vi "GUI.vi"() -> ()   [LabVIEW 2015]
doc: "The myRIO Project template acquires acceleration data from the onboard accelerometer and displays the changes of acceleration values in a waveform chart."
uses:
  Labview/Kinect Project/Kinect Project/subVIs/Log Level Control.ctl
  Labview/Kinect Project/Kinect Project/subVIs/Video Resolution Control.ctl
  Labview/Kinect Project/Kinect Project/subVIs/Video Format Control.ctl
  Labview/Kinect Project/Kinect Project/subVIs/Depth Format Control.ctl
  Labview/Kinect Project/Kinect Project/subVIs/Depth Resolution Control.ctl
  Labview/Kinect Project/Kinect Project/subVIs/Led Control.ctl
panel:
  out "Start angle":dbl
  in  "Ring":u16(ring)
  out "Hazard location":dbl[](array[numeric])
  out "# of targets chosen":dbl
  out "Tab indicator":string
  in  "Map Displays":enum32{"Display map", "Obsticle map"}(tab)
  out "Display map":u16[][](array[ring])
  in  "Obsticle map":u16[][](array[ring])
  in  "Robot information":enum32{"Robot info", "Status updates"}(tab)
  out "Paused LED":bool
  out "Robot angle":dbl
  out "Robot location (grid)":dbl[](array[numeric])
  out "Target location":dbl[](array[numeric])
  out "Route":dbl[][](array[numeric])
  out "Robot location (cm)":dbl[](array[numeric])
  in  "Pause":bool
  in  "stop":bool
  out "Map key words":string[](array[string])
  out "Map key":u16[](array[ring])
  out "Waitning for user input LED":bool
  out "Executing route LED":bool
  out "Slecting target LED":bool
  out "Altering amp LED":bool
  out "Scanning LED":bool
  out "Initializing LED":bool
  in  "Options and instructions":T1(tab)
  out "Initialize map LED":bool
  in  "Robot starting angle":dbl
  in  "Robot starting location":dbl[](array[numeric])
  in  "Load":bool
  in  "Start":bool
  in  "Angle to scan around":dbl
  in  "Scan or move toggle":bool
  in  "Start scan or move button":bool
  out "Scan or move":bool
  in  "Run auto correct":bool
  out "Auto correct Led":bool
  in  "Alter map button":bool
  out "Alter map LED":bool
  out "To many targets":bool
  in  "Chose location button":bool
  in  "Chose location switch":bool
  out "Calulated target location":dbl[](array[numeric])
  out "Chose location LED":bool
  out "Kinect Handle":i64
  out "Video Handle out":i64
  out "Object location":dbl[][](array[numeric])
  out "p":dbl
  out "Centre location":dbl[](array[numeric])
  out "Map dimensions":dbl[](array[numeric])
  # "The text on the left indicates which \ntab you should be on"
  # "On the right is the robots location on the grid and\nin cm from the top left corner of the map"
  # "The angle the robot is facing is displayed on the right. An angle of 0 \nis relative to north on the map, 90 is east, 180 is south and 270 is west"
  # "The destiniation on the grid that the robot is trying to reach is \ndisplayed in the box Target location and the route it will take \ndisplayed in Route"
  # "If you wish to stop the program from running press the button in\nthe top right of the screen or the button to the right. To pause the \nprogram after its current task use the toggle switch to the left"
  # "When paused light will be on"
  # "The lights below indicate what task the \nrobot is currently completing"
  # "Below is the key for the map"
  # "Initializing"
  # "Scanning for hazards and obsticles"
  # "Altering map"
  # "Selecting target location"
  # "Executing route"
  # "Waiting for user input"
  # "When this light is on you will need to select the initilization mode"
  # "Use the switch on the left to select wether you want to start from a new \npredefined map or wether you want to start from the last saved map. It is \nkey that if conection was lost and restablished that you start from loading \nthe last saved map"
  # "If you are starting from the a new map type in the starting location of \nthe robot. Remeber that the angle is relative to NSEW on the map with \nan angle of 0 being North"
  # "Once you are happy with your selection press the start button to the left \nto start the robot moving."
  # "When this light is on you can choose wether to move to another \npoint or scan at the robots current location"
  # "Using the toggle switch to the right you will be able to chose \nwether you want to scan 180 degree around the robots current \nloation after which you can adjust the map and chose the next \nlocation to move to or wether you would like the robot just move \nto a location before which you can alter the map if need be"
  # "If you decide to scan you can alter the angle that the DaNI will scan\naround. The angle will be defaulted to the DaNI's current location"
  # "Once you are have decided on wether to move or scan using \nthe toggle swtich, press the button on the right to select your \nchosen option"
  # "When this light is on you will be able to alter the map for any errors.\nYou can manualy make changes but this should only be done at this \nstage and on the obsticle map"
  # "If you would like the program to run an autocorrect on the map press\nthe button to the right. If the green light is on autocorrect is running \nso don't change anything on the map as it will not be saved."
  # "Once you are happy with the changes press the button on the left and\nthe changes will be saved and the program will continue executing"
  # "When this light is on you will need to select the location to use.\nIf the light on the right flashes too many or not enough locations\nwhere selected"
  # "Use this screen to decide wether to use the target location calulated \nby the program or select your own target location. Once the taget \nlocation has been set a route will be calulated and the robot will \nmove to this location"
  # "Use the switch on the left to select wether to use the calculated\nlocation or use your own. To select your own select it on the map \nby changing the square Dark blue. Only select one square or it will \nnot be accepted"
  # "Once you are happy with the chosen location press the button \non the left to continue"
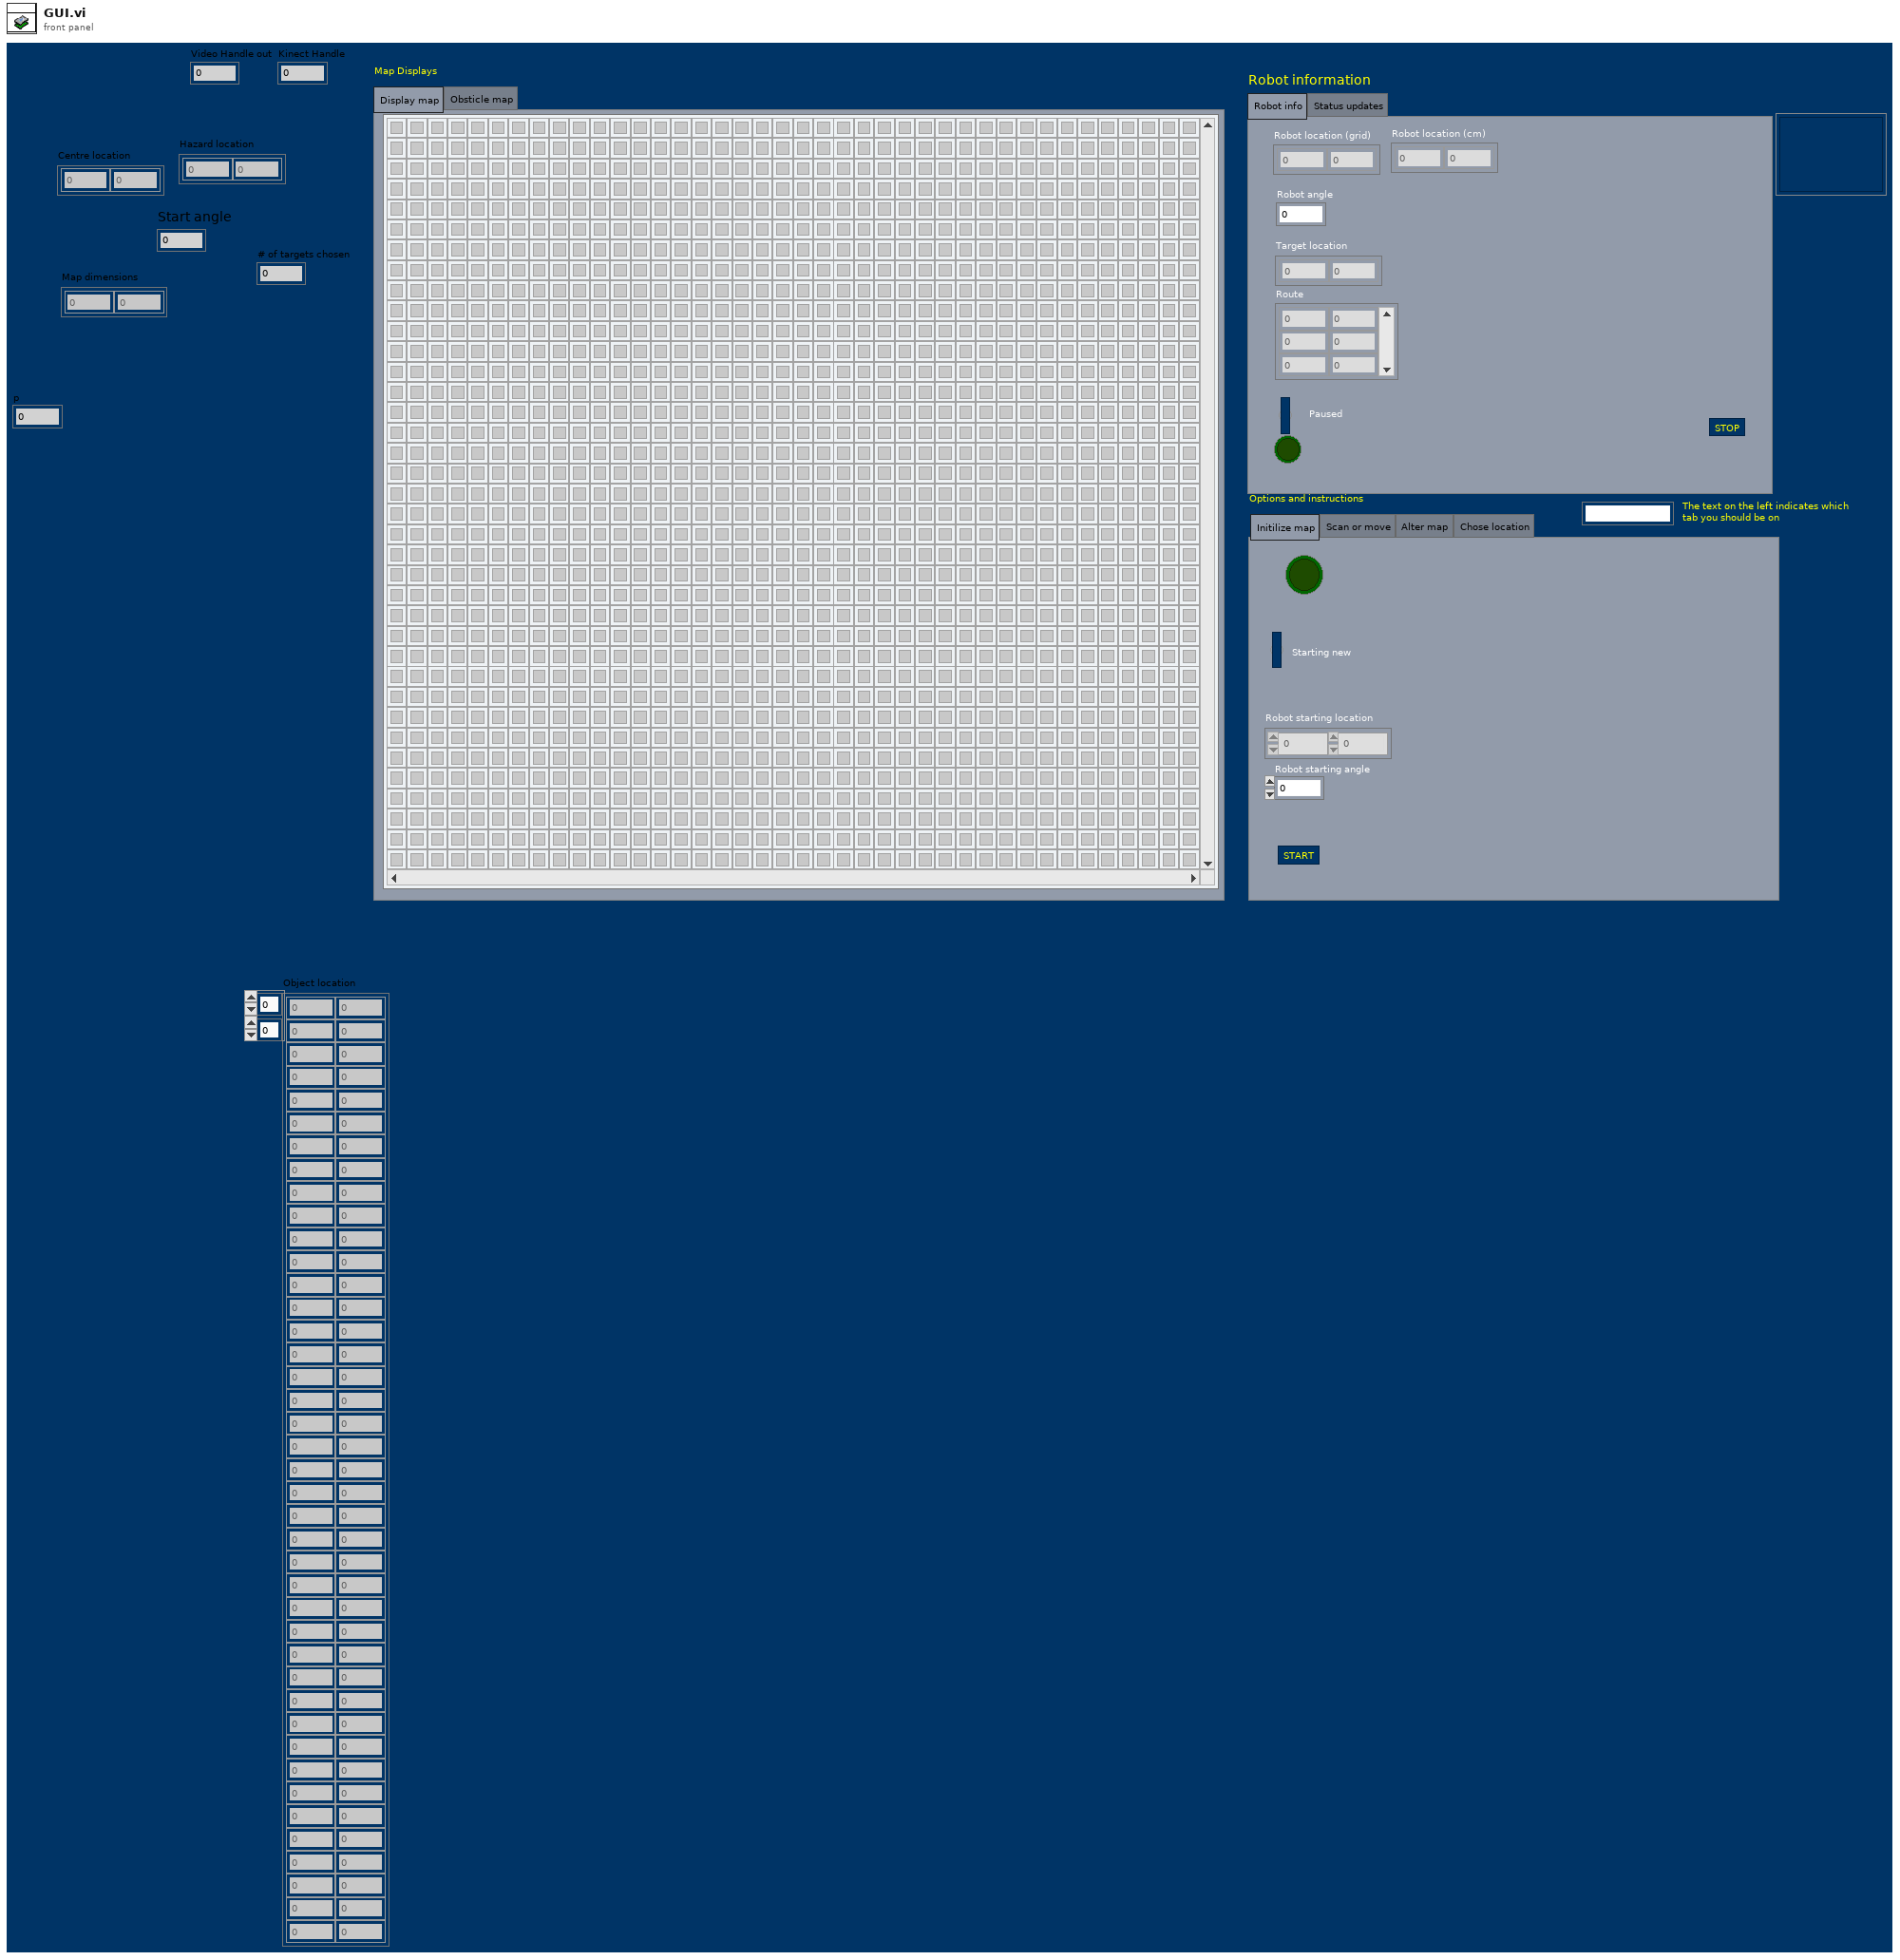
[diagram p1: front panel]
types:
  T1 = enum32{"Initilize map", "Scan or move", "Alter map", "Chose location"}
  T2 = typedef "Led Control.ctl" = enum32{"LED_OFF", "LED_GREEN", "LED_RED", "LED_YELLOW", "LED_BLINK_GREEN", "LED_BLINK_GREEN2", "LED_BLINK_RED_YELLOW"}
  T3 = typedef "Video Resolution Control.ctl" = enum32{"FREENECT_RESOLUTION_LOW", "FREENECT_RESOLUTION_MEDIUM", "FREENECT_RESOLUTION_HIGH"}
  T4 = typedef "Video Format Control.ctl" = enum32{"FREENECT_VIDEO_RGB", "FREENECT_VIDEO_BAYER", "FREENECT_VIDEO_IR_8BIT", "FREENECT_VIDEO_IR_10BIT", "FREENECT_VIDEO_IR_10BIT_PACKED", "FREENECT_VIDEO_YUV_RGB", "FREENECT_VIDEO_YUV_RAW"}
  T5 = typedef "Depth Format Control.ctl" = enum32{"FREENECT_DEPTH_11BIT", "FREENECT_DEPTH_10BIT", "FREENECT_DEPTH_11BIT_PACKED", "FREENECT_DEPTH_10BIT_PACKED", "FREENECT_DEPTH_REGISTERED", "FREENECT_DEPTH_MM"}
  T6 = typedef "Depth Resolution Control.ctl" = enum16{"FREENECT_RESOLUTION_TINY", "FREENECT_RESOLUTION_LOW", "FREENECT_RESOLUTION_MEDIUM"}
  T7 = cluster{"Video Resolution":T3, "Video Format":T4, "Depth Format":T5, "Depth Resolution":T6}
  T8 = typedef "Log Level Control.ctl" = enum32{"FREENECT_LOG_FATAL", "FREENECT_LOG_ERROR", "FREENECT_LOG_WARNING", "FREENECT_LOG_NOTICE", "FREENECT_LOG_INFO", "FREENECT_LOG_DEBUG", "FREENECT_LOG_SPEW", "FREENECT_LOG_FLOOD"}
  T9 = cluster{"Hue Range":cluster{"Lower value":i32, "Upper value":i32}, "Sat Range":cluster{"Lower value":i32, "Upper value":i32}, "Luma Range":cluster{"Lower value":i32, "Upper value":i32}}
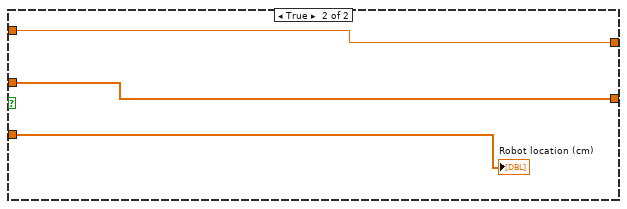
[diagram p2: hidden frame]
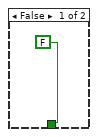
[diagram p5: hidden frame]
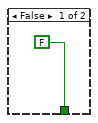
[diagram p6: hidden frame]
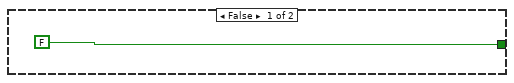
[diagram p8: hidden frame]
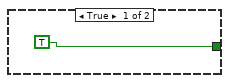
[diagram p9: hidden frame]
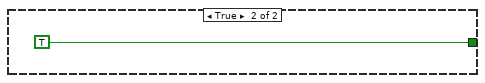
[diagram p10: hidden frame]
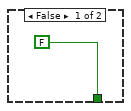
[diagram p12: hidden frame]
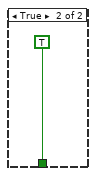
[diagram p13: hidden frame]
diagram:
  n1 = flat-sequence {
    frame #0 {
      n2 = flat-sequence {
        tunnel: [w7] -> w2
        tunnel: [w7] -> w1
        tunnel: w2 -> [w15]
        tunnel: w1 -> [w14]
        frame #0 {
          w3 = FALSE
          n3 = local write "Waitning for user input LED"(w3) -> ()
          n4 = local write "Executing route LED"(w3) -> ()
          n5 = local write "Initializing LED"(w3) -> ()
          n6 = local write "Paused LED"(w3) -> ()
          n7 = local write "Altering amp LED"(w3) -> ()
          n8 = local write "Slecting target LED"(w3) -> ()
          n9 = local write "Scanning LED"(w3) -> ()
          "Map key" <- i32[] [0, 1, 2, 4, 6, 3, 7, 8, 5]
          "Map key words" <- string[] ["Empty area", "Obsticle", "Unexplored area", "Robot location", "Robots front", "Target location", "Route", "Hazard", "Black box"]
        }
        frame #1 {
          w6 = FALSE
          n10 = while {
            tunnel: ["Load"] -> w7
            stop <- "Start" stop-if-true
            w10 = TRUE
            "Tab indicator" <- "Initialize map tab"
            "Initialize map LED" <- w10
            "Initializing LED" <- w10
          }
          n11 = local write "Auto correct Led"(w6) -> ()
          n12 = local write "Chose location LED"(w6) -> ()
          n13 = local write "Alter map LED"(w6) -> ()
          n14 = local write "Robot location (cm)"(dbl[] [0.0, 0.0]) -> ()
          n15 = local write "Route"(i32[][] []) -> ()
          n16 = local write "Scan or move"(w6) -> ()
        }
        frame #2 {
          n17 = call "Inizialize map.vi"("Boolean"=w14) -> ("Map dimesions"=→"Map dimensions":dbl[], "Map initialize"=w17:dbl[][], "Robot start location"=w18:dbl[], "Robot actual location"=w20:dbl[], "Robot angle"=w22:dbl)  [unwired: 6 in]
          n18 = local write "Obsticle map"(w17) -> ()
          n19 = case shown="False" w15 {
            tunnel: w18 -> [_ w43]
            tunnel: ["Robot starting location" w43] -> w19
            tunnel: w20 -> [_ w41]
            tunnel: ["Robot starting angle" w42] -> w21
            tunnel: w22 -> [_ w42]
            frame False {
              w30 = 2.5
              w35 = 5
              n20 = Index Array(array="Robot starting location", index #1=0, index #2=1) -> (element #1=w37:dbl, element #2=w36:dbl)
              n21 = Multiply(x=w37, y=w35) -> (x*y=w33:dbl)
              n22 = Multiply(x=w36, y=w35) -> (x*y=w34:dbl)
              n23 = Add(x=w33, y=w30) -> (x+y=w25:dbl)
              n24 = Add(x=w34, y=w30) -> (x+y=w26:dbl)
              n25 = local read "Robot location (cm)"() -> (w27:dbl[])
              n26 = Replace Array Subset(array=w27, new element #1=w25, index #1=0, new element #2=w26, index #2=1) -> (w28:dbl[])
              n27 = local write "Robot location (cm)"(w28) -> ()
            }
            frame True {
              "Robot location (cm)" <- w41
            }
          }
          "Robot location (grid)" <- w19
          "Robot angle" <- w21
          n28 = local write "Initialize map LED"(FALSE) -> ()
          n29 = local write "Tab indicator"("Any") -> ()
        }
        frame #3 {
          n30 = call "Initialize IMU.vi"() -> ()  [unwired: 12 in]
          n31 = call "LED control.vi"("RED/green"="Green") -> ()  [unwired: 11 in]
        }
        frame #4 {
          n32 = call "Initialize kinect systems.vi"("Video and Depth config"=T7 {"Video Resolution"=enum."FREENECT_RESOLUTION_MEDIUM", "Video Format"=enum."FREENECT_VIDEO_RGB", "Depth Format"=enum."FREENECT_DEPTH_11BIT", "Depth Resolution"=enum."FREENECT_RESOLUTION_LOW"} ("Video & Depth Config"), "Led Option"=Led_Control."LED_OFF", "tilt degree"=-15 ("Tilt degree"), "Log Level"=Log_Level_Control."FREENECT_LOG_FATAL") -> ("Kinect Handle"=→"Kinect Handle":i64, "Video Handle out"=→"Video Handle out":i64)  [unwired: 4 in, 2 out]
        }
        frame #5 {
          n33 = local read "Robot location (cm)"() -> (w53:dbl[])
          n34 = local read "Robot angle"() -> (w54:dbl)
          n35 = local read "Obsticle map"() -> (w52:u16[][])
          n36 = call "Update robot location and direction.vi"("Map input"=w52, "Actual robot location"=w53, "Robot angle"=w54) -> ("Map Output"=→"Display map":dbl[][], "Centre location"=→"Centre location":dbl[])  [unwired: 6 in]
          n37 = local write "Initializing LED"(FALSE) -> ()
        }
        frame #6 {
          n38 = while {
            stop <- w57 stop-if-true
            n39 = local read "Pause"() -> (w57:bool)
            n40 = local write "Paused LED"(TRUE) -> ()
          }
        }
      }
    }
    frame #1 {
      n41 = while {
        stop <- "stop" stop-if-true
        n42 = flat-sequence {
          tunnel: [w63] -> w60
          tunnel: w60 -> [w72]
          tunnel: [w72] -> w59
          tunnel: w59 -> [w74]
          frame #0 {
            n43 = local read "Robot angle"() -> (w62:dbl)
            n44 = local write "Angle to scan around"(w62) -> ()
          }
          frame #1 {
            n45 = while {
              tunnel: ["Scan or move toggle"] -> w63
              stop <- "Start scan or move button" stop-if-true
              n46 = local write "Paused LED"(FALSE) -> ()
              n47 = local write "Tab indicator"("Scan or move") -> ()
              n48 = call "LED control.vi"("RED/green"="Red") -> ()  [unwired: 11 in]
              "Scan or move" <- TRUE
              "Waitning for user input LED" <- TRUE
            }
          }
          frame #2 {
            n49 = call "LED control.vi"("RED/green"="Green") -> ()  [unwired: 11 in]
          }
          frame #3 {
            w73 = FALSE
            n50 = case shown="True" w74 {
              frame False {
              }
              frame True {
                n51 = flat-sequence {
                  frame #0 {
                    n52 = local read "Robot angle"() -> (w77:dbl)
                    n53 = call "Turning control.vi"("Robot angle"=w77, "Angle to move to"="Angle to scan around") -> ("Final Robot angle"=w76:dbl)  [unwired: 8 in]
                    n54 = local write "Angle to scan around"(w76) -> ()
                  }
                  frame #1 {
                    n55 = local read "Robot angle"() -> (w81:dbl)
                    n56 = call "correct angle.vi"("Robot angle"=w81, "Angle moved"=-90.0) -> ("Final angle"=w80:dbl)  [unwired: 9 in]
                    n57 = call "Turning control.vi"("Robot angle"=w81, "Angle to move to"=w80) -> ("Final Robot angle"=w79:dbl)  [unwired: 8 in]
                    "Start angle" <- w79
                    n58 = local write "Robot angle"(w79) -> ()
                    "Scanning LED" <- TRUE
                  }
                  frame #2 {
                    n59 = while {
                      stop <- w84 stop-if-true
                      n60 = flat-sequence {
                        tunnel: [w93] -> w87
                        tunnel: w87 -> [w94]
                        tunnel: [w94] -> w86
                        tunnel: w86 -> [w97]
                        tunnel: [w102] -> w88
                        tunnel: w88 -> [w108]
                        tunnel: [w113] -> _
                        tunnel: [w113] -> w85
                        tunnel: w85 -> [w121]
                        tunnel: [w122] -> w84
                        frame #0 {
                          n61 = local read "Robot location (cm)"() -> (w92:dbl[])
                          n62 = local read "Robot angle"() -> (w93:dbl)
                          n63 = call "Kinect Depth Controler.vi"("Angle"=w93, "Robot Location"=w92) -> ("p"=→"p":dbl, "Object location"=→"Object location":dbl[][])  [unwired: 7 in, 1 out]
                          n64 = local write "Paused LED"(FALSE) -> ()
                        }
                        frame #1 {
                        }
                        frame #2 {
                          n65 = local read "Obsticle map"() -> (w96:u16[][])
                          n66 = local read "Object location"() -> (w95:dbl[][])
                          n67 = local read "Robot location (grid)"() -> (w99:dbl[])
                          n68 = local read "p"() -> (w98:dbl)
                          n69 = call "Update obsticles.vi"("angle input"=w97, "Robot Location"=w99, "p"=w98, "Map Input"=w96, "Object location"=w95) -> ("Map output"=w100:dbl[][])  [unwired: 6 in]
                          n70 = local write "Obsticle map"(w100) -> ()
                        }
                        frame #3 {
                          n71 = local read "Robot location (cm)"() -> (w106:dbl[])
                          n72 = local read "Robot angle"() -> (w105:dbl)
                          n73 = call "Kinect Video Controller.vi"("HSL Ranges"=T9 {"Hue Range"={"Lower value"=200, "Upper value"=254}, "Sat Range"={"Lower value"=190, "Upper value"=254}, "Luma Range"={"Lower value"=0, "Upper value"=140}}, "Robot angle"=w105, "robot location"=w106) -> ("y"=w103:dbl, "x"=w101:dbl, "Hazard location"=→"Hazard location":dbl[])  [unwired: 6 in]
                          n74 = call "Validate hazard.vi"("y"=w103, "x"=w101) -> ("Valid"=w102:bool)  [unwired: 9 in]
                        }
                        frame #4 {
                          n75 = case shown="True" w108 {
                            frame False {
                            }
                            frame True {
                              n76 = local read "Obsticle map"() -> (w111:u16[][])
                              n77 = local read "Hazard location"() -> (w110:dbl[])
                              n78 = call "Update Hazards.vi"("Map Input"=w111, "Hazard location"=w110) -> ("Map Output"=w109:dbl[][])  [unwired: 9 in]
                              n79 = local write "Obsticle map"(w109) -> ()
                            }
                          }
                        }
                        frame #5 {
                          n80 = local read "Robot angle"() -> (w114:dbl)
                          n81 = call "turning.vi"("Turn time"=110, "clock anticlock"="Clock") -> ("angle moved"=w115:dbl)  [unwired: 9 in]
                          n82 = call "correct angle.vi"("Robot angle"=w114, "Angle moved"=w115) -> ("Final angle"=w113:dbl)  [unwired: 9 in]
                          n83 = local write "Robot angle"(w113) -> ()
                        }
                        frame #6 {
                          w117 = 5
                          n84 = local read "Start angle"() -> (w126:dbl)
                          n85 = call "correct angle.vi"("Robot angle"=w126, "Angle moved"=180) -> ("Final angle"=w120:dbl)  [unwired: 9 in]
                          n86 = Add(x=w120, y=w117) -> (x+y=w119:dbl)
                          n87 = Subtract(x=w120, y=w117) -> (x-y=w118:dbl)
                          n88 = Less Or Equal?(x=w121, y=w119) -> (x <= y?=w123:bool)
                          n89 = Greater Or Equal?(x=w121, y=w118) -> (x >= y?=w124:bool)
                          n90 = case shown="True" w124 {
                            tunnel: w123 -> [_ w129]
                            tunnel: [FALSE w128] -> w122
                            frame False {
                            }
                            frame True {
                              n91 = case shown="True" w129 {
                                tunnel: [FALSE TRUE] -> w128
                                frame False {
                                }
                                frame True {
                                }
                              }
                            }
                          }
                        }
                        frame #7 {
                          n92 = while {
                            stop <- w132 stop-if-true
                            n93 = local read "Pause"() -> (w132:bool)
                            n94 = local write "Paused LED"(FALSE) -> ()
                          }
                        }
                      }
                    }
                  }
                  frame #3 {
                    n95 = local read "Robot angle"() -> (w135:dbl)
                    n96 = call "correct angle.vi"("Robot angle"=w135, "Angle moved"=-90.0) -> ("Final angle"=w136:dbl)  [unwired: 9 in]
                    n97 = call "Turning control.vi"("Robot angle"=w135, "Angle to move to"=w136) -> ("Final Robot angle"=w134:dbl)  [unwired: 8 in]
                    n98 = local write "Robot angle"(w134) -> ()
                  }
                }
              }
            }
            n99 = local write "Scan or move"(w73) -> ()
            n100 = local write "Waitning for user input LED"(w73) -> ()
            n101 = local write "Tab indicator"("Any") -> ()
          }
          frame #4 {
            n102 = local read "Robot location (cm)"() -> (w142:dbl[])
            n103 = local read "Map dimensions"() -> (w139:dbl[])
            n104 = local read "Obsticle map"() -> (w143:u16[][])
            n105 = local read "Robot angle"() -> (w141:dbl)
            n106 = local write "Scanning LED"(FALSE) -> ()
            n107 = call "Save data.vi"("file path (use dialog)"=path "/home/lvuser/natinst/bin/DaNIdata.txt", "Obsticle map"=w143, "Robot angle"=w141, "Actual robot location"=w142, "Map dimensions"=w139) -> ()  [unwired: 7 in]
          }
          frame #5 {
            n108 = while {
              stop <- "Alter map button" stop-if-true
              w144 = TRUE
              n109 = flat-sequence {
                frame #0 {
                  # "add in revert code vi"
                }
                frame #1 {
                  n110 = case shown="True" "Run auto correct" {
                    frame False {
                    }
                    frame True {
                      n111 = flat-sequence {
                        frame #0 {
                          n112 = local read "Map dimensions"() -> (w151:dbl[])
                          n113 = local read "Obsticle map"() -> (w150:u16[][])
                          n114 = call "correct map.vi"("Map dimensions"=w151, "Obsticle map"=w150) -> ("Corrected map"=w149:u16[][])  [unwired: 9 in]
                          n115 = local write "Obsticle map"(w149) -> ()
                          "Auto correct Led" <- TRUE
                        }
                        frame #1 {
                          n116 = Wait (ms)(milliseconds to wait=1000) -> ()  [unwired: 1 out]
                        }
                      }
                    }
                  }
                }
                frame #2 {
                  n117 = local write "Auto correct Led"(FALSE) -> ()
                }
              }
              n118 = local write "Tab indicator"("Alter map") -> ()
              n119 = local write "Waitning for user input LED"(w144) -> ()
              "Alter map LED" <- w144
              "Altering amp LED" <- w144
            }
          }
          frame #6 {
            w154 = FALSE
            n120 = local read "Robot location (cm)"() -> (w156:dbl[])
            n121 = local read "Obsticle map"() -> (w157:u16[][])
            n122 = local read "Robot angle"() -> (w155:dbl)
            n123 = local write "Alter map LED"(w154) -> ()
            n124 = local write "Waitning for user input LED"(w154) -> ()
            n125 = call "Update robot location and direction.vi"("Map input"=w157, "Actual robot location"=w156, "Robot angle"=w155) -> ("Map Output"=w158:dbl[][], "Centre location"=w159:dbl[])  [unwired: 6 in]
            n126 = local write "Display map"(w158) -> ()
            n127 = local write "Centre location"(w159) -> ()
          }
          frame #7 {
            n128 = local read "Display map"() -> (w162:u16[][])
            n129 = local read "Robot location (grid)"() -> (w161:dbl[])
            n130 = local write "Tab indicator"("Any") -> ()
            n131 = call "Improved find target.vi"("robot location"=w161, "Dispaly map"=w162) -> ("target location"=→"Target location" →"Calulated target location":dbl[])  [unwired: 8 in]
          }
          frame #8 {
            n132 = local read "Target location"() -> (w165:dbl[])
            n133 = local read "Display map"() -> (w166:u16[][])
            n134 = local read "Route"() -> (w167:dbl[][])
            n135 = call "Update route + target location.vi"("Route"=w167, "Map input"=w166, "Target Location"=w165) -> ("Map Output"=w164:dbl[][])  [unwired: 8 in]
            n136 = local write "Display map"(w164) -> ()
          }
          frame #9 {
            n137 = while {
              stop <- w172 stop-if-true
              w169 = TRUE
              n138 = local write "To many targets"(FALSE) -> ()
              n139 = case shown="True" "Chose location button" {
                tunnel: "Chose location switch" -> [_ w178]
                tunnel: [FALSE w177] -> w172
                frame False {
                }
                frame True {
                  n140 = case shown="False" w178 {
                    tunnel: [w182 TRUE] -> w177
                    frame False {
                      # "add in find target location"
                      n141 = local read "Map dimensions"() -> (w184:dbl[])
                      n142 = local read "Obsticle map"() -> (w185:u16[][])
                      n143 = call "Find choosen target.vi"("Map dimensions"=w184, "Display map"=w185) -> ("Numeric"=w181:dbl, "Target location"=w183:dbl[])  [unwired: 8 in]
                      "# of targets chosen" <- w181
                      n144 = local write "Target location"(w183) -> ()
                      n145 = Equal?(x=w181, y=1) -> (x = y?=w179:bool)
                      n146 = case shown="False" w179 {
                        tunnel: [TRUE w188] -> w182
                        frame True {
                        }
                        frame False {
                          n147 = flat-sequence {
                            tunnel: [FALSE] -> w187
                            tunnel: [w192] -> w188
                            tunnel: w187 -> [w192]
                            frame #0 {
                            }
                            frame #1 {
                              n148 = Wait (ms)(milliseconds to wait=1000) -> ()  [unwired: 1 out]
                              "To many targets" <- TRUE
                            }
                          }
                        }
                      }
                    }
                    frame True {
                    }
                  }
                }
              }
              n149 = local write "Waitning for user input LED"(w169) -> ()
              n150 = local write "Tab indicator"("Choose location") -> ()
              n151 = local write "Altering amp LED"(FALSE) -> ()
              "Chose location LED" <- TRUE
              "Slecting target LED" <- w169
            }
          }
          frame #10 {
            w194 = FALSE
            n152 = local read "Target location"() -> (w202:dbl[])
            n153 = local read "Obsticle map"() -> (w199:u16[][])
            n154 = local write "Waitning for user input LED"(w194) -> ()
            n155 = local write "Chose location LED"(w194) -> ()
            n156 = Index Array(array=w202, index #1=0, index #2=1) -> (element #1=w196:dbl, element #2=w197:dbl)
            n157 = Replace Array Subset(array=w199, new element=0, index (row)=w197, index (col)=w196) -> (w198:u16[][])
            n158 = local write "Obsticle map"(w198) -> ()
          }
          frame #11 {
            n159 = local read "Map dimensions"() -> (w206:dbl[])
            n160 = local read "Display map"() -> (w207:u16[][])
            n161 = local read "Target location"() -> (w205:dbl[])
            n162 = local read "Centre location"() -> (w204:dbl[])
            n163 = local write "Tab indicator"("Any") -> ()
            n164 = call "Choose route.vi"("robot location"=w204, "target location"=w205, "Map dimensions"=w206, "Map"=w207) -> ("Route"=→"Route":dbl[][])  [unwired: 7 in]
          }
          frame #12 {
            n165 = local read "Target location"() -> (w211:dbl[])
            n166 = local read "Display map"() -> (w210:u16[][])
            n167 = local read "Route"() -> (w209:dbl[][])
            n168 = call "Update route + target location.vi"("Route"=w209, "Map input"=w210, "Target Location"=w211) -> ("Map Output"=w212:dbl[][])  [unwired: 8 in]
            n169 = local write "Display map"(w212) -> ()
          }
          frame #13 {
            n170 = while {
              stop <- w215 stop-if-true
              n171 = flat-sequence {
                tunnel: [w218] -> w216
                tunnel: w216 -> [w226]
                tunnel: [w239] -> w215
                frame #0 {
                  n172 = local read "Robot location (grid)"() -> (w221:dbl[])
                  n173 = local read "Robot location (cm)"() -> (w223:dbl[])
                  n174 = local read "Robot angle"() -> (w222:dbl)
                  n175 = local read "Route"() -> (w224:dbl[][])
                  n176 = call "Execute Route.vi"("Robot location"=w221, "Robot angle"=w222, "Actual robot location"=w223, "Route"=w224) -> ("Succesful movemnet"=w218:bool, "New grid robot location"=w225:dbl[], "New angle"=w220:dbl, "New actaul robot location"=w219:dbl[])  [unwired: 4 in]
                  n177 = local write "Paused LED"(FALSE) -> ()
                  n178 = local write "Robot location (grid)"(w225) -> ()
                  n179 = local write "Robot location (cm)"(w219) -> ()
                  n180 = local write "Robot angle"(w220) -> ()
                }
                frame #1 {
                  n181 = case shown="True" w226 {
                    frame False {
                    }
                    frame True {
                      n182 = local read "Route"() -> (w229:dbl[][])
                      n183 = Delete From Array(array=w229, index (row)=0) -> (array with subset deleted=w227:dbl[][])  [unwired: 2 in, 1 out]
                      n184 = local write "Route"(w227) -> ()
                    }
                  }
                }
                frame #2 {
                  n185 = local read "Robot location (cm)"() -> (w231:dbl[])
                  n186 = local read "Obsticle map"() -> (w232:u16[][])
                  n187 = local read "Robot angle"() -> (w230:dbl)
                  n188 = call "Update robot location and direction.vi"("Map input"=w232, "Actual robot location"=w231, "Robot angle"=w230) -> ("Map Output"=w234:dbl[][], "Centre location"=w233:dbl[])  [unwired: 6 in]
                  n189 = local write "Centre location"(w233) -> ()
                  n190 = local write "Display map"(w234) -> ()
                }
                frame #3 {
                  n191 = local read "Target location"() -> (w238:dbl[])
                  n192 = local read "Display map"() -> (w237:u16[][])
                  n193 = local read "Route"() -> (w236:dbl[][])
                  n194 = call "Update route + target location.vi"("Route"=w236, "Map input"=w237, "Target Location"=w238) -> ("Map Output"=w235:dbl[][])  [unwired: 8 in]
                  n195 = local write "Display map"(w235) -> ()
                }
                frame #4 {
                  w246 = 1
                  w247 = 0
                  n196 = local read "Target location"() -> (w248:dbl[])
                  n197 = local read "Centre location"() -> (w249:dbl[])
                  n198 = Index Array(array=w248, index #1=w247, index #2=w246) -> (element #1=w245:dbl, element #2=w243:dbl)
                  n199 = Index Array(array=w249, index #1=w247, index #2=w246) -> (element #1=w244:dbl, element #2=w242:dbl)
                  n200 = Equal?(x=w243, y=w242) -> (x = y?=w241:bool)
                  n201 = Equal?(x=w245, y=w244) -> (x = y?=w240:bool)
                  n202 = case shown="True" w241 {
                    tunnel: w240 -> [_ w252]
                    tunnel: [FALSE w251] -> w239
                    frame False {
                    }
                    frame True {
                      n203 = case shown="False" w252 {
                        tunnel: [FALSE TRUE] -> w251
                        frame False {
                        }
                        frame True {
                        }
                      }
                    }
                  }
                }
                frame #5 {
                  n204 = while {
                    stop <- "Pause" stop-if-true
                    "Paused LED" <- TRUE
                  }
                }
              }
              n205 = local write "Slecting target LED"(FALSE) -> ()
              "Executing route LED" <- TRUE
            }
          }
          frame #14 {
            n206 = local write "Executing route LED"(FALSE) -> ()
          }
        }
      }
    }
    frame #2 {
      n207 = local read "Video Handle out"() -> (w258:i64)
      n208 = local read "Kinect Handle"() -> (w259:i64)
      n209 = call "Close kinect systems.vi"("Kinect Handle"=w259, "Video handle in"=w258) -> ()  [unwired: 9 in, 1 out]
    }
  }
